vi "LoadDatabase.vi"() -> (1 "Deispersion compenastion factor":dbl, 2 "Refractive index":dbl, 3 "Glass name":string)   [LabVIEW 2013]
panel:
  in  "x":bool
  in  "stop":bool
  out "Result Set":string[][](table) caption="Result Set (from first statement with results)"
  in  "OK Button":bool
  in  "Multicolumn Listbox":i32(listbox)
  in  "DatabaseList":string(combo)
  out "db_name":string
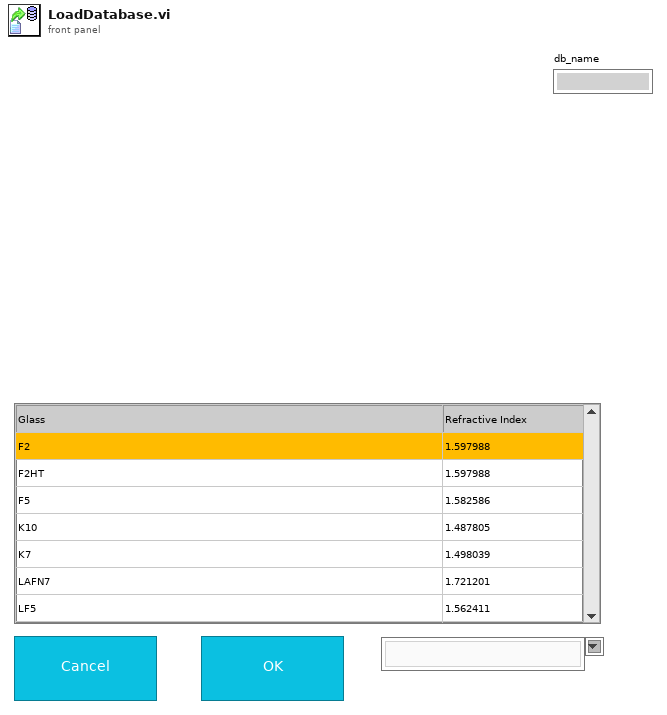
[diagram p1: front panel]
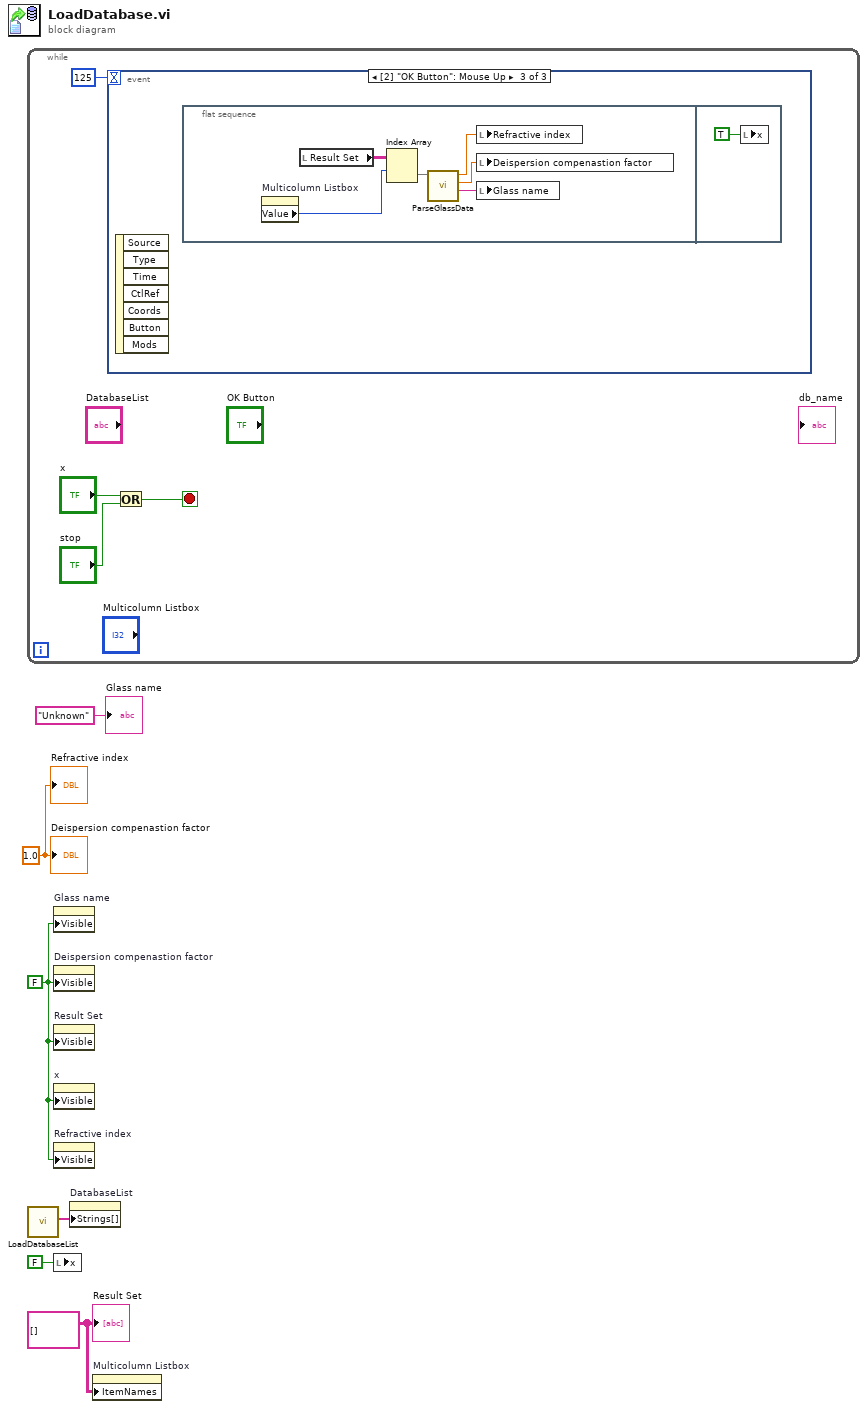
[diagram p0: block diagram]
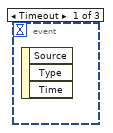
[diagram p2: hidden frame]
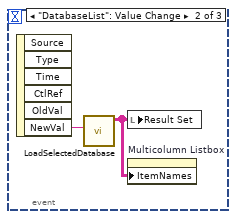
[diagram p3: hidden frame]
diagram:
  w1 = 1.0 ("Refractive index")
  w3 = FALSE ("Visible")
  w5 = string[][] [] ("Result Set")
  n1 = while {
    stop <- w8 stop-if-true
    n2 = event shown="[2] \"OK Button\": Mouse Up" {
      selector: _ -> [_ _ _]
      dyn-events: _ -> [_ _ _]
      timeout: 125 -> [_ _ _]
      event Timeout {
        n3 = event-data() -> ()  [unwired: 1 in, 3 out]
      }
      event "DatabaseList": Value Change {
        n4 = event-data() -> ("NewVal"=w12:string)  [unwired: 1 in, 5 out]
        n5 = call "LoadSelectedDatabase.vi"("Value"=w12) -> ("Result Set"=w11:string[][])  [unwired: 10 in]
        n6 = local write "Result Set"(w11) -> ()
        n7 = property on="Multicolumn Listbox" class="MCListbox (strict)"("ItemNames"=w11) -> ()  [unwired: 2 in, 2 out]
      }
      event "OK Button": Mouse Up {
        n8 = event-data() -> ()  [unwired: 1 in, 7 out]
        n9 = flat-sequence {
          frame #0 {
            n10 = property on="Multicolumn Listbox" class="MCListbox (strict)"() -> ("Value"=w14:i32)  [unwired: 2 in, 2 out]
            n11 = local read "Result Set"() -> (w13:string[][])
            n12 = Index Array(array=w13, index (row)=w14) -> (element=w15:string[])  [unwired: 1 in]
            n13 = call "ParseGlassData.vi"("Result Set"=w15) -> ("String"=w16:string, "Numeric"=w18:dbl, "Numeric 2"=w17:dbl)  [unwired: 8 in]
            n14 = local write "Refractive index"(w17) -> ()
            n15 = local write "Deispersion compenastion factor"(w18) -> ()
            n16 = local write "Glass name"(w16) -> ()
          }
          frame #1 {
            n17 = local write "x"(TRUE ("stop")) -> ()
          }
        }
      }
    }
    n18 = Or(x="x", y="stop") -> (x .or. y?=w8:bool)
  }
  n19 = call "LoadDatabaseList.vi"() -> ("filenames"=w6:string[])  [unwired: 9 in, 2 out]
  n20 = property on="Glass name" class="Str"("Visible"=w3) -> ()  [unwired: 2 in, 2 out]
  n21 = property on="Deispersion compenastion factor" class="DigNum (strict)"("Visible"=w3) -> ()  [unwired: 2 in, 2 out]
  n22 = property on="Result Set" class="Tbl (strict)"("Visible"=w3) -> ()  [unwired: 2 in, 2 out]
  n23 = property on="x" class="Bool (strict)"("Visible"=w3) -> ()  [unwired: 2 in, 2 out]
  n24 = property on="Refractive index" class="DigNum (strict)"("Visible"=w3) -> ()  [unwired: 2 in, 2 out]
  n25 = local write "x"(FALSE ("x")) -> ()
  n26 = property on="DatabaseList" class="CmbBox"("Strings[]"=w6) -> ()  [unwired: 2 in, 2 out]
  n27 = property on="Multicolumn Listbox" class="MCListbox (strict)"("ItemNames"=w5) -> ()  [unwired: 2 in, 2 out]
  "Result Set" <- w5
  "Deispersion compenastion factor" <- w1
  "Refractive index" <- w1
  "Glass name" <- "Unknown" ("Glass name")
